vi "Game_CanBuyAVowel.vi"(8 "error in (no error)":errorcluster, 10 "player":T1, 11 "Players array":T2[](array[typedef])) -> (0 "error out":errorcluster, 1 "CanBuy?":bool, 2 "player OUT":T1, 3 "Players array OUT":T2[](array[typedef]))   [LabVIEW 2020]
uses:
  Typedefs/enumeratedPlayers.ctl
  Typedefs/game_player.ctl
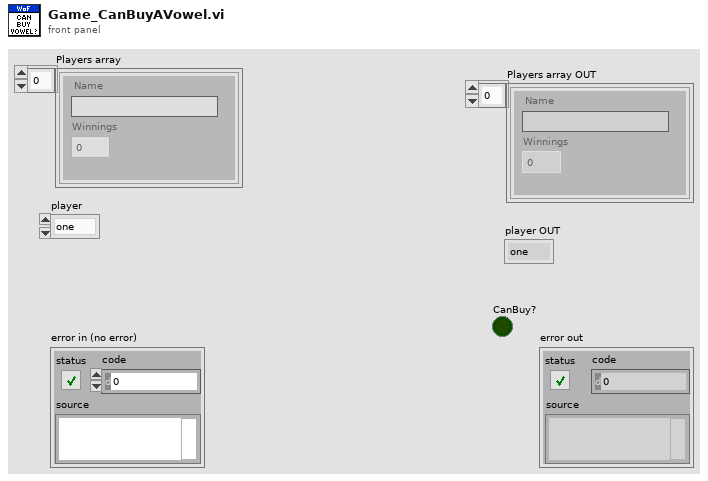
[diagram p1: front panel]
types:
  T1 = typedef "enumeratedPlayers.ctl" = enum16{"one", "two", "three"}
  T2 = typedef "game_player.ctl" = cluster{"Name":string, "Winnings":dbl}
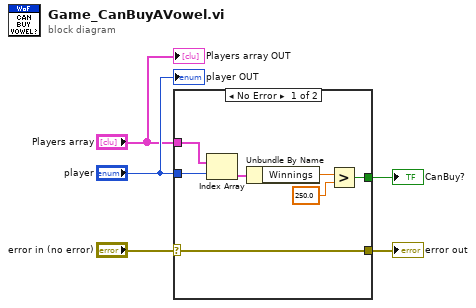
[diagram p0: block diagram]
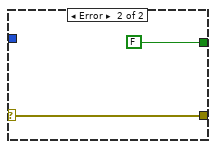
[diagram p2: hidden frame]
diagram:
  n1 = case shown="No Error" "error in (no error)" {
    selector: "error in (no error)" -> [w6 w14]
    tunnel: "player" -> [w11 _]
    tunnel: "Players array" -> [w12 _]
    tunnel: [w7 FALSE] -> w2
    tunnel: [w6 w14] -> w1
    frame No Error {
      n2 = Index Array(array=w12, index=w11) -> (element=w10:T2)
      n3 = Unbundle By Name(w10) -> ("Winnings"=w9:dbl)
      n4 = Greater?(x=w9, y=250.0) -> (0:w7:bool)
    }
    frame Error {
    }
  }
  "error out" <- w1
  "CanBuy?" <- w2
  "Players array OUT" <- "Players array"
  "player OUT" <- "player"
